vi "NewPhotonCounterBig.vi"(8 "error in":errorcluster) -> (0 "error out":errorcluster, 3 "task out":refnum<k21>)   [LabVIEW 2015]
uses:
  <vilib>/DAQmx/configure/timing.llb/DAQmx Timing (Sample Clock).vi
  <vilib>/DAQmx/create/channels.llb/DAQmx Create Channel (AI-Voltage-Basic).vi
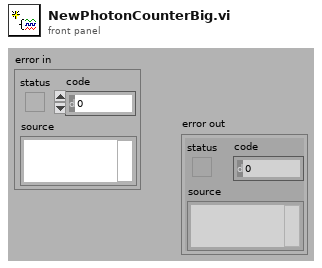
[diagram p1: front panel]
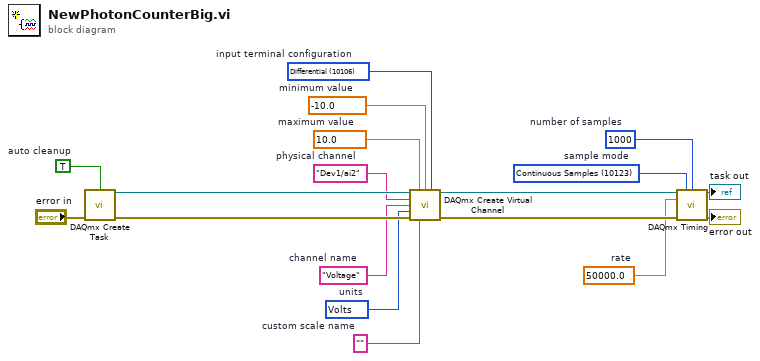
[diagram p0: block diagram]
diagram:
  w1 = 10123 items=["Finite Samples"=10178, "Continuous Samples"=10123, "Hardware Timed Single Point"=12522]  # sample mode
  w2 = 1000  # number of samples
  w3 = 50000.0  # rate
  w7 = 10106 items=["default"=-1, "RSE"=10083, "NRSE"=10078, "Differential"=10106, "Pseudodifferential"=12529]  # input terminal configuration
  w8 = 10348 items=["Volts"=10348, "From Custom Scale"=10065]  # units
  w9 = "Voltage"  # channel name
  w11 = ""  # custom scale name
  w12 = -10.0  # minimum value
  w13 = 10.0  # maximum value
  w14 = "Dev1/ai2"  # physical channel
  w16 = TRUE  # auto cleanup
  n1 = call <vilib>:"DAQmx Create Task.vi"("auto cleanup"=w16, "error in"="error in") -> ("task out"=w15:refnum<k21>, "error out"=w17:errorcluster)  [unwired: 12 in]
  n2 = call-poly <vilib>:"DAQmx Create Virtual Channel.vi"("task in"=w15, "maximum value"=w13, "minimum value"=w12, "input terminal configuration"=w7, "physical channels"=w14, "name to assign"=w9, "units"=w8, "error in"=w17, "custom scale name"=w11) -> ("task out"=w4:refnum<k21>, "error out"=w10:errorcluster)  [unwired: 5 in]
  n3 = call-poly <vilib>:"DAQmx Timing.vi"("task/channels in"=w4, "sample mode"=w1, "samples per channel"=w2, "rate"=w3, "error in"=w10) -> ("task out"=→"task out":refnum<k21>, "error out"=→"error out":errorcluster)  [unwired: 9 in]
